vi "AlliGator Get Phasor Ratio Map Color v2.vi"(6 "Image Display Palette Information":T2 {"Palette Type" items=["Grayscale", "Binary", "Gradient", "Rainbow", "Temperature", "User Defined", "Binary 16 Bit", "Gradient 16 Bit", "Rainbow 16 Bit", "Temperature 16 Bit", "User Defined 16 Bit"]}, 7 "Color Fading?":bool, 8 "Error In":errorcluster, 9 "Phasor Ratio Display Range":cluster{"Min":dbl, "Max":dbl}={"Min"=0.0, "Max"=1.0}, 10 "-d_0":sgl, 11 "Phasor Ratio Data":T1) -> (0 "Error Out":errorcluster, 1 "Transparent?":bool, 3 "Overlay Color":T4)   [LabVIEW 2021, in "AlliGator Phasor Ratio.lvlib"]
doc: "Computes phasor ratio equivalent color using the provided color scale."
uses:
  AlliGator Phasor Ratio.lvlib
  Palette/Image Palette Information.ctl
  Image/Image Display Palette Type.ctl
  AlliGator Phasor Ratio Data.ctl
  <vilib>/vision/NI_Vision_Development_Module.lvlib
  Image/Image.lvlib
  Palette/Palette.lvlib
panel:
  # "see the AlliGator License on the block diagram (Ctrl+E or Window:Show Block Diagram)"
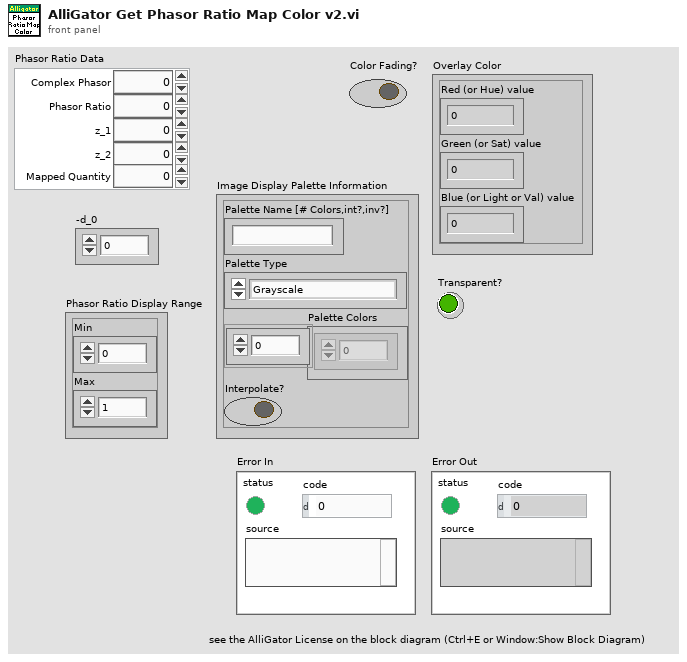
[diagram p1: front panel]
types:
  T1 = typedef "AlliGator Phasor Ratio.lvlib/AlliGator Phasor Ratio Data.ctl" = cluster{"Complex Phasor":csg, "Phasor Ratio":sgl, "z_1":csg, "z_2":csg, "Mapped Quantity":sgl}
  T2 = typedef "Palette.lvlib/Image Palette Information.ctl" = cluster{"Palette Name [# Colors,int?,inv?]":string, "Palette Type":T3, "Palette Colors":u32[], "Interpolate?":bool}
  T3 = typedef "Image.lvlib/Image Display Palette Type.ctl" = u32
  T4 = cluster{"Red (or Hue) value":u8, "Green (or Sat) value":u8, "Blue (or Light or Val) value":u8}
  T5 = cluster{"Red (or Hue) value":u8, "Green (or Sat) value":u8, "Blue (or Light or Val) value":u8}[]
  T6 = cluster{"Red (or Hue) value":sgl, "Green (or Sat) value":sgl, "Blue (or Light or Val) value":sgl}
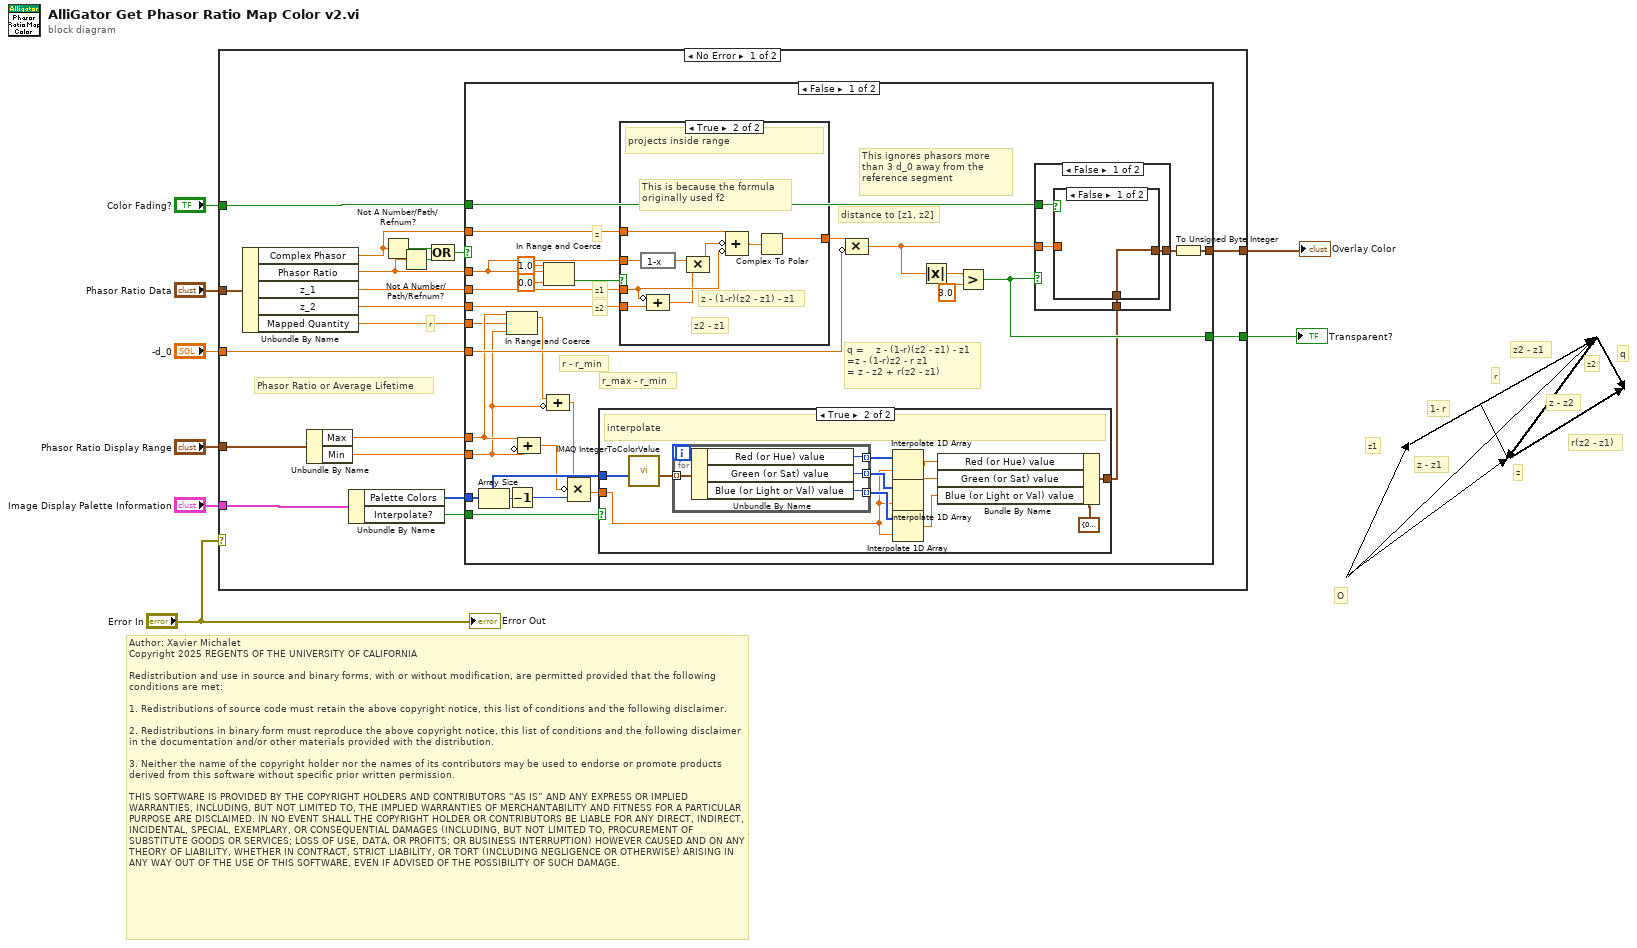
[diagram p0: block diagram]
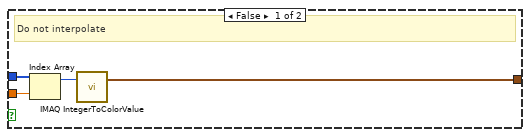
[diagram p2: hidden frame]
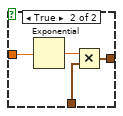
[diagram p3: hidden frame]
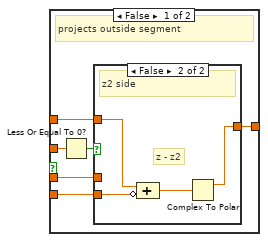
[diagram p5: hidden frame]
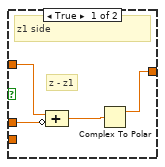
[diagram p6: hidden frame]
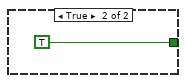
[diagram p7: hidden frame]
diagram:
  # "Author: Xavier Michalet\nCopyright 2025 REGENTS OF THE UNIVERSITY OF CALIFORNIA\n\nRedistribution and use in source and binary forms, with or without modification, are permitted provided that the following conditions are met:\n\n1. Redistributions of source code must retain the above copyright notice, this list of conditions and the following disclaimer.\n\n2. Redistributions in binary form must reproduce the above copyright notice, this list of conditions and the following disclaimer in the documentation and/or other materials provided with the distribution.\n\n3. Neither the name of the copyright holder nor the names of its contributors may be used to endorse or promote products derived from this software without specific prior written permission.\n\nTHIS SOFTWARE IS PROVIDED BY THE COPYRIGHT HOLDERS AND CONTRIBUTORS “AS IS” AND ANY EXPRESS OR IMPLIED WARRANTIES, INCLUDING, BUT NOT LIMITED TO, THE IMPLIED WARRANTIES OF MERCHANTABILITY AND FITNESS FOR A PARTICULAR PURPOSE ARE DISCLAIMED. IN NO EVENT SHALL THE COPYRIGHT HOLDER OR CONTRIBUTORS BE LIABLE FOR ANY DIRECT, INDIRECT, INCIDENTAL, SPECIAL, EXEMPLARY, OR CONSEQUENTIAL DAMAGES (INCLUDING, BUT NOT LIMITED TO, PROCUREMENT OF SUBSTITUTE GOODS OR SERVICES; LOSS OF USE, DATA, OR PROFITS; OR BUSINESS INTERRUPTION) HOWEVER CAUSED AND ON ANY THEORY OF LIABILITY, WHETHER IN CONTRACT, STRICT LIABILITY, OR TORT (INCLUDING NEGLIGENCE OR OTHERWISE) ARISING IN ANY WAY OUT OF THE USE OF THIS SOFTWARE, EVEN IF ADVISED OF THE POSSIBILITY OF SUCH DAMAGE."
  # "O"
  # "q"
  # "r(z2 - z1)"
  # "1- r"
  # "r"
  # "z - z2"
  # "z - z1"
  # "z2 - z1"
  # "z"
  # "z2"
  # "z1"
  n1 = case shown="No Error" "Error In" {
    tunnel: "-d_0" -> [w27 _]
    tunnel: [w26 _] -> w7
    tunnel: [w25 _] -> w6
    tunnel: "Color Fading?" -> [w24 _]
    tunnel: "Image Display Palette Information" -> [w20 _]
    tunnel: "Phasor Ratio Data" -> [w17 _]
    tunnel: "Phasor Ratio Display Range" -> [w12 _]
    frame No Error {
      # "r"
      # "Phasor Ratio or Average Lifetime"
      n2 = Unbundle By Name(w17) -> ("Complex Phasor"=w16:csg, "Phasor Ratio"=w15:sgl, "z_1"=w14:csg, "z_2"=w13:csg, "Mapped Quantity"=w9:sgl)
      n3 = Unbundle By Name(w12) -> ("Max"=w11:dbl, "Min"=w10:dbl)
      n4 = Unbundle By Name(w20) -> ("Palette Colors"=w19:u32[], "Interpolate?"=w18:bool)
      n5 = Not A Number/Path/Refnum?(number/path/refnum=w16) -> (NaN/Path/Refnum?=w23:bool)
      n6 = Not A Number/Path/Refnum?(number/path/refnum=w15) -> (NaN/Path/Refnum?=w22:bool)
      n7 = Compound Arithmetic op=OR(w23, w22) -> (w21:bool)
      n8 = case shown="False" w21 {
        tunnel: w14 -> [w55 _]
        tunnel: w13 -> [w54 _]
        tunnel: w27 -> [w52 _]
        tunnel: [w35 _] -> w26
        tunnel: [w50 TRUE] -> w25
        tunnel: w24 -> [w49 _]
        tunnel: w16 -> [w48 _]
        tunnel: w15 -> [w34 _]
        tunnel: w19 -> [w43 _]
        tunnel: w18 -> [w44 _]
        tunnel: w11 -> [w40 _]
        tunnel: w10 -> [w38 _]
        tunnel: w9 -> [w36 _]
        frame False {
          # "distance to [z1, z2]"
          # "q =    z - (1-r)(z2 - z1) - z1\n=z - (1-r)z2 - r z1\n= z - z2 + r(z2 - z1)"
          # "z"
          # "z2"
          # "z1"
          # "r_max - r_min"
          # "r - r_min"
          # "This ignores phasors more than 3 d_0 away from the reference segment"
          n9 = Array Size(array=w43) -> (size(s)=w47:i32)
          n10 = In Range and Coerce(upper limit=w40, x=w36, lower limit=w38) -> (coerced(x)=w46:dbl)  [unwired: 1 out]
          n11 = Decrement(x=w47) -> (x-1=w45:i32)
          n12 = Compound Arithmetic op=ADD(w40, invert w38) -> (w39:dbl)
          n13 = In Range and Coerce(upper limit=sgl 1.0, x=w34, lower limit=sgl 0.0) -> (In Range?=w33:bool)  [unwired: 1 out]
          n14 = Compound Arithmetic op=ADD(w46, invert w38) -> (w37:dbl)
          n15 = Compound Arithmetic op=MULTIPLY(w37, invert w39, w45) -> (w42:dbl)
          n16 = case shown="True" w44 {
            tunnel: w43 -> [w59 w70]
            tunnel: w42 -> [w58 w65]
            tunnel: [w56 w60] -> w41
            frame False {
              # "Do not interpolate"
              n17 = Index Array(array=w59, index=w58) -> (element=w57:u32)
              n18 = call "IMAQ IntegerToColorValue"("U32 value"=w57) -> ("Color Value"=w56:T4)  [unwired: 4 in, 3 out]
            }
            frame True {
              # "interpolate"
              n19 = call "IMAQ IntegerToColorValue"("1D U32 array"=w70) -> ("1D Color value array"=w69:T5)  [unwired: 4 in, 3 out]
              n20 = for {
                tunnel: w69 -> [w74] mode=indexing
                tunnel: [w73] -> w68 mode=indexing
                tunnel: [w72] -> w67 mode=indexing
                tunnel: [w71] -> w66 mode=indexing
                n21 = Unbundle By Name(w74) -> ("Red (or Hue) value"=w73:u8, "Green (or Sat) value"=w72:u8, "Blue (or Light or Val) value"=w71:u8)
              }
              n22 = Interpolate 1D Array(1:w65, 2:w68) -> (0:w63:dbl)
              n23 = Interpolate 1D Array(1:w65, 2:w67) -> (0:w62:dbl)
              n24 = Interpolate 1D Array(1:w65, 2:w66) -> (0:w61:dbl)
              n25 = Bundle By Name(cluster=T4 {"Red (or Hue) value"=0, "Green (or Sat) value"=0, "Blue (or Light or Val) value"=0} ("input cluster"), "Red (or Hue) value"=w63, "Green (or Sat) value"=w62, "Blue (or Light or Val) value"=w61) -> (w60:T4)
            }
          }
          n26 = case shown="True" w33 {
            tunnel: w48 -> [w87 w106]
            tunnel: w55 -> [w86 w100]
            tunnel: w34 -> [w89 w105]
            tunnel: [w85 w102] -> w53
            tunnel: w54 -> [w84 w101]
            frame False {
              # "projects outside segment"
              n27 = Less Or Equal To 0?(x=w89) -> (x <= 0?=w88:bool)
              n28 = case shown="False" w88 {
                tunnel: w87 -> [w93 w97]
                tunnel: w86 -> [w92 _]
                tunnel: [w90 w95] -> w85
                tunnel: w84 -> [_ w94]
                frame True {
                  # "z - z1"
                  # "z1 side"
                  n29 = Compound Arithmetic op=ADD(w93, invert w92) -> (w91:csg)
                  n30 = Complex To Polar(r * e^(i*theta)=w91) -> (r=w90:sgl)  [unwired: 1 out]
                }
                frame False {
                  # "z - z2"
                  # "z2 side"
                  n31 = Compound Arithmetic op=ADD(w97, invert w94) -> (w96:csg)
                  n32 = Complex To Polar(r * e^(i*theta)=w96) -> (r=w95:sgl)  [unwired: 1 out]
                }
              }
            }
            frame True {
              # "z - (1-r)(z2 - z1) - z1"
              # "z2 - z1"
              # "This is because the formula originally used f2"
              # "projects inside range"
              n33 = expression code="1-x"(w105) -> (w98:sgl)
              n34 = Compound Arithmetic op=ADD(invert w100, w101) -> (w99:csg)
              n35 = Compound Arithmetic op=MULTIPLY(w98, w99) -> (w104:csg)
              n36 = Compound Arithmetic op=ADD(w106, invert w104, invert w100) -> (w103:csg)
              n37 = Complex To Polar(r * e^(i*theta)=w103) -> (r=w102:sgl)  [unwired: 1 out]
            }
          }
          n38 = Compound Arithmetic op=MULTIPLY(w53, invert w52) -> (w30:sgl)
          n39 = Absolute Value(x=w30) -> (abs(x)=w29:sgl)
          n40 = Greater?(x=w29, y=sgl 3.0) -> (0:w50:bool)
          n41 = case shown="False" w50 {
            tunnel: w41 -> [w78 _]
            tunnel: w30 -> [w77 _]
            tunnel: [w76 _] -> w51
            tunnel: w49 -> [w75 _]
            frame False {
              n42 = case shown="False" w75 {
                tunnel: w78 -> [w79 w83]
                tunnel: w77 -> [_ w81]
                tunnel: [w79 w80] -> w76
                frame False {
                }
                frame True {
                  n43 = Exponential(1:w81) -> (0:w82:sgl)
                  n44 = Multiply(x=w82, y=w83) -> (x*y=w80:T6)
                }
              }
            }
            frame True {
            }
          }
          n45 = To Unsigned Byte Integer(number=w51) -> (unsigned 8bit integer=w35:T4)
        }
        frame True {
        }
      }
    }
    frame Error {
    }
  }
  "Overlay Color" <- w7
  "Transparent?" <- w6
  "Error Out" <- "Error In"
